vi "Logger File Create.vi"(8 "error in":errorcluster, 9 "Test Stand Name":string, 10 "Project Base Path":path, 11 "Logger in":refnum<class "Logger.lvclass">) -> (0 "error out":errorcluster, 3 "Logger out":refnum<class "Logger.lvclass">)   [LabVIEW 2019, in "TS Framework.lvlib" / "Logger.lvclass"]
uses:
  Logger.lvclass
  Logger.lvclass/Logger.ctl
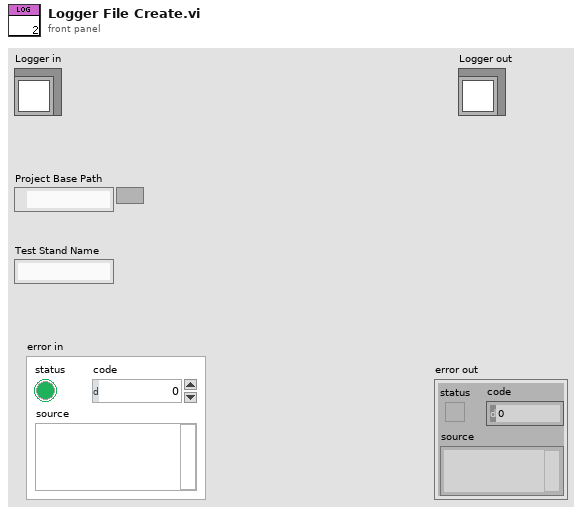
[diagram p1: front panel]
types:
  T1 = enum16{"open", "replace", "create", "open or create", "replace or create", "replace or create with confirmation"}
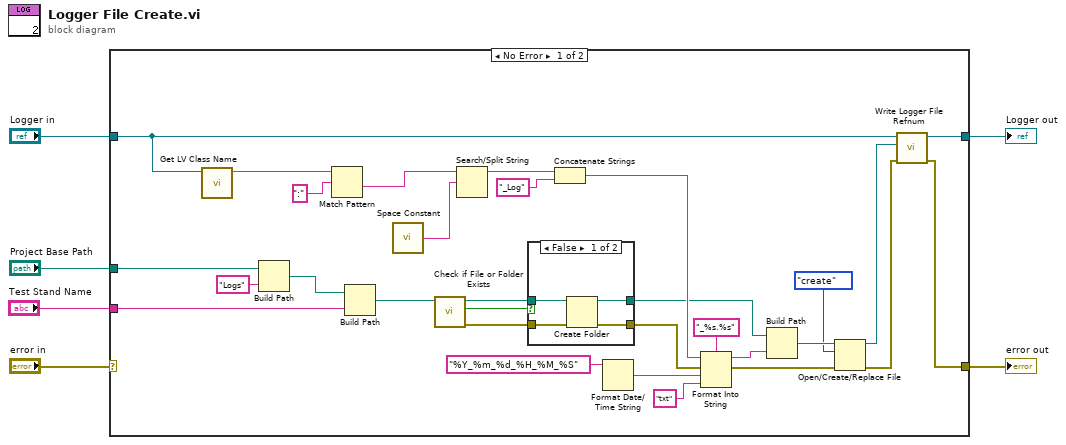
[diagram p0: block diagram]
diagram:
  n1 = case shown="No Error" "error in" {
    selector: "error in" -> [_ w44]
    tunnel: "Project Base Path" -> [w7 _]
    tunnel: [w15 w44] -> w3
    tunnel: "Logger in" -> [w18 w43]
    tunnel: [w14 w43] -> w2
    tunnel: "Test Stand Name" -> [w9 _]
    frame No Error {
      n2 = call <vilib>:"Get LV Class Name.vi"("object"=w18) -> ("class name"=w13:string)  [unwired: 9 in, 1 out]
      n3 = Build Path(base path=w7, name or relative path="Logs") -> (appended path=w10:path)
      n4 = Match Pattern(string=w13, regular expression=":") -> (after substring=w11:string)  [unwired: 1 in, 3 out]
      n5 = Build Path(base path=w10, name or relative path=w9) -> (appended path=w8:path)
      n6 = call <vilib>:"Space Constant.vi"() -> ("String"=w31:string)
      n7 = call <vilib>:"Check if File or Folder Exists.vi"("path"=w8) -> ("error out"=w34:errorcluster, "file or folder exists?"=w36:bool, "dup path"=w35:path)  [unwired: 8 in]
      n8 = Search/Split String(string=w11, search string/char (-)=w31) -> (substring before match=w32:string)  [unwired: 1 in, 2 out]
      n9 = case shown="False" w36 {
        tunnel: w35 -> [w40 w42]
        tunnel: w34 -> [w39 w41]
        tunnel: [w37 w42] -> w19
        tunnel: [w38 w41] -> w20
        frame False {
          n10 = Create Folder(path (use dialog)=w40, error in=w39) -> (created path=w37:path, error out=w38:errorcluster)  [unwired: 1 in, 1 out]
        }
        frame True {
        }
      }
      n11 = Concatenate Strings(w32, "_Log" ("string")) -> (w21:string)
      n12 = Format Date/Time String(time format string (%c)="%Y_%m_%d_%H_%M_%S") -> (date/time string=w27:string)  [unwired: 2 in]
      n13 = Format Into String(format string="_%s.%s", initial string=w21, error in=w20, w27, "txt" ("input 2")) -> (resulting string=w26:string, error out=w23:errorcluster)
      n14 = Build Path(base path=w19, name or relative path=w26) -> (appended path=w25:path)
      n15 = Open/Create/Replace File(file path (use dialog)=w25, error in=w23, operation (0:open)=T1."create") -> (refnum out=w17:refnum<file>, error out=w16:errorcluster)  [unwired: 3 in, 1 out]
      n16 = call "Write Logger File Refnum.vi"("error in (no error)"=w16, "Logger File Refnum"=w17, "Logger in"=w18) -> ("error out"=w15:errorcluster, "Logger out"=w14:refnum<class "Logger.lvclass">)  [unwired: 7 in]
    }
    frame Error {
    }
  }
  "error out" <- w3
  "Logger out" <- w2
